vi "SPI Write Read N Frames.vi"(5 "CS Configuration":T1, 7 "SPI Channel (0)":u8, 8 "Error In":errorcluster, 9 "SPI Frame Size (0)":u8, 10 "Data":u8[](array[numeric]), 11 "LINX Resource":T3) -> (0 "Error Out":errorcluster, 1 "Read Data":u8[](array[numeric]), 3 "LINX Resource":T3)   [LabVIEW 2011, in "LVH-LINX.lvlib"]
doc: "Write/Read the specified SPI channel. SPI is full duplex, therefore the write and read operations take place simultaneously.\n\n<b>SPI Channel</b> specifies the device SPI channel to write/read to.\n\n<b>Data</b> is a U8 array of data bytes to shift out starting with Data[0] to Data[n-1].\n\n<b>SPI Frame Size</b> determinse the number of bytes shifted out between toggling CS.\n\n<b>CS Channel</b> is the Chip Select (DIO) channel to use during the SPI transaction.\n\n<b>CS Logic Level</b> specifies the logic level of the CS pin. Active low is most common and means that CS will idle high, then be driven low when a frame begins. The number of bytes specified in SPI Frame Size will be transfered, then CS will be driven high to end the frame. This process is repeated until all bytes in Data have been shifted out."
uses:
  LVH-LINX.lvlib
  Private/Type Defs/LINX Ref.ctl
  Private/Type Defs/Platform.ctl
  Private/Type Defs/Interface.ctl
  Private/Device/Type Defs/LINX Device Config.ctl
  Private/Device/Type Defs/TCP Config.ctl
  Private/Device/Type Defs/Channels.ctl
  SPI CS Config.ctl
  Private/Type Defs/Peripherals/SPI/SPI CS Logic Level.ctl
  Private/Type Defs/Peripheral.ctl
  Private/Type Defs/Channel FGV States.ctl
  Private/Device/Device.lvlib
  <vilib>/myRIO/Common/Instrument Driver Framework/myRIO v1.0/SPI/typedefs/SPI Frame Length.ctl
  <vilib>/myRIO/Common/Instrument Driver Framework/myRIO v1.0/SPI/typedefs/SPI Data Direction.ctl
  <vilib>/myRIO/Common/Instrument Driver Framework/myRIO v1.0/SPI/typedefs/SPI Clock Polarity.ctl
  <vilib>/LabVIEW Hacker/LINX/Private/Type Defs/Peripherals/SPI/SPI Clock Phase.ctl
  <vilib>/myRIO/Instrument Drivers/Onboard IO/SPI/typedefs/SPI Configuration.ctl
  <vilib>/myRIO/Common/Instrument Driver Framework/myRIO v1.0/SPI/typedefs/SPI Channels Enum.ctl
  <vilib>/myRIO/Common/Instrument Driver Framework/Utilities/typedefs/Generic FPGA Reference.ctl
  <vilib>/myRIO/Common/Instrument Driver Framework/Utilities/typedefs/myRIO v1.0 Reference.ctl
  <vilib>/myRIO/Common/Instrument Driver Framework/Utilities/typedefs/Hardware Version Enum.ctl
  <vilib>/myRIO/Common/Instrument Driver Framework/Utilities/typedefs/myRIO Generic Hardware Reference.ctl
  <vilib>/myRIO/Instrument Drivers/Onboard IO/SPI/typedefs/SPI Reference.ctl
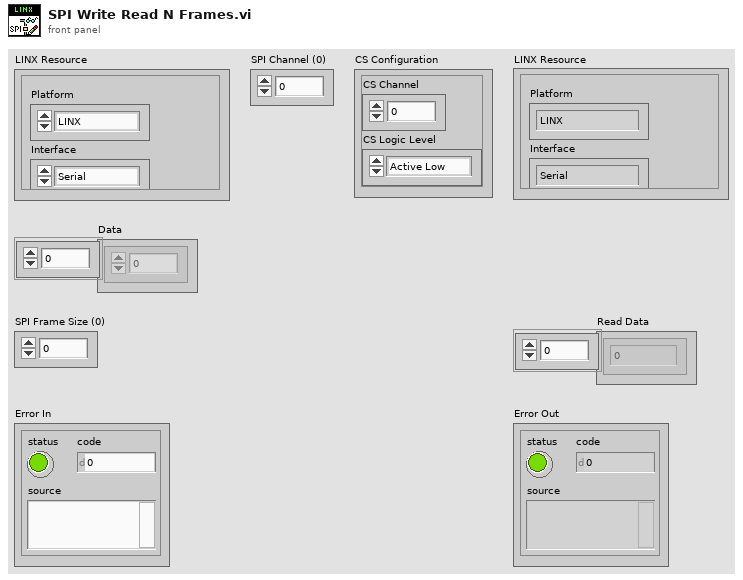
[diagram p1: front panel]
types:
  T1 = typedef "LVH-LINX.lvlib/SPI CS Config.ctl" = cluster{"CS Channel":u8, "CS Logic Level":T2}
  T2 = typedef "LVH-LINX.lvlib/SPI CS Logic Level.ctl" = enum8{"Active Low", "Active High"}
  T3 = typedef "LVH-LINX.lvlib/LINX Ref.ctl" = cluster{"Platform":T4, "Interface":T5, "LINX Device Config":T6}
  T4 = typedef "LVH-LINX.lvlib/Platform.ctl" = enum16{"LINX", "myRIO"}
  T5 = typedef "LVH-LINX.lvlib/Interface.ctl" = enum16{"Serial", "TCP"}
  T6 = typedef "LVH-LINX.lvlib/Device.lvlib/LINX Device Config.ctl" = cluster{"Interface":T5, "COM Port":refnum<visa-resource-name>, "TCP Configuration":T7, "Device Family":u8, "Device ID":u8, "Device Name":string, "TCP Ref":refnum<k5>, "Channels":T8}
  T7 = typedef "LVH-LINX.lvlib/Device.lvlib/TCP Config.ctl" = cluster{"IP Address":string, "Port":u16}
  T8 = typedef "LVH-LINX.lvlib/Channels.ctl" = cluster{"DI Channels":u8[], "DO Channels":u8[], "AI":u8[], "AO":u8[], "PWM":u8[], "QE":u8[], "UART":u8[], "I2C 2":u8[], "SPI":u8[], "CAN":u8[], "AI Ref (V)":dbl, "AO Resolution (Bits)":u8, "AO Ref (V)":dbl}
  T9 = typedef "LVH-LINX.lvlib/Peripheral.ctl" = enum8{"DI", "DO", "AI", "AO", "PWM", "QE", "UART", "I2C", "SPI", "CAN"}
  T10 = typedef "LVH-LINX.lvlib/Channel FGV States.ctl" = enum16{"Initialize", "Get", "Set"}
  T11 = typedef "SPI.lvlib/SPI Reference.ctl" = cluster{"myRIO Reference":T12, "SPI Channels Enum":T16, "SPI Configuration":T17}
  T12 = typedef "myRIO Generic Hardware Reference.ctl" = cluster{"myRIO Model":T13, "myRIO Hardware Reference":T14}
  T13 = typedef "Hardware Version Enum.ctl" = enum16{"Unknown", "myRIO-1900", "myRIO-1950"}
  T14 = typedef "myRIO v1.0 Reference.ctl" = cluster{"Generic FPGA Reference":T15, "Allow multiple opens":bool}
  T15 = typedef "Generic FPGA Reference.ctl" = refnum<k20>
  T16 = typedef "SPI Channels Enum.ctl" = enum16{"Not Connected", "A/SPI", "B/SPI"}
  T17 = typedef "SPI.lvlib/SPI Configuration.ctl" = cluster{"Frequency (Hz)":dbl, "Clock Phase":T18, "Clock Polarity":T19, "Data Direction":T20, "Frame Length":T21}
  T18 = typedef "LVH-LINX.lvlib/SPI Clock Phase.ctl" = enum8{"Leading", "Trailing"}
  T19 = typedef "SPI Clock Polarity.ctl" = enum8{"Low", "High"}
  T20 = typedef "SPI Data Direction.ctl" = enum8{"Most Significant Bit First", "Least Significant Bit First"}
  T21 = typedef "SPI Frame Length.ctl" = u8
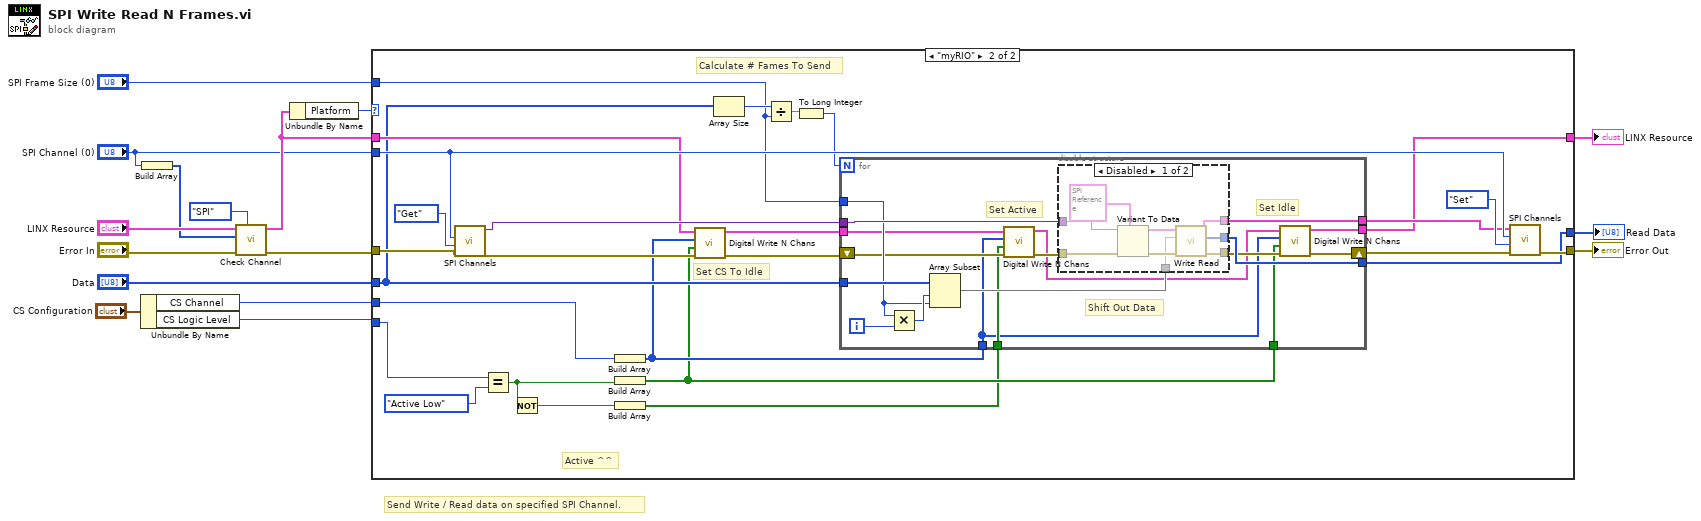
[diagram p0: block diagram]
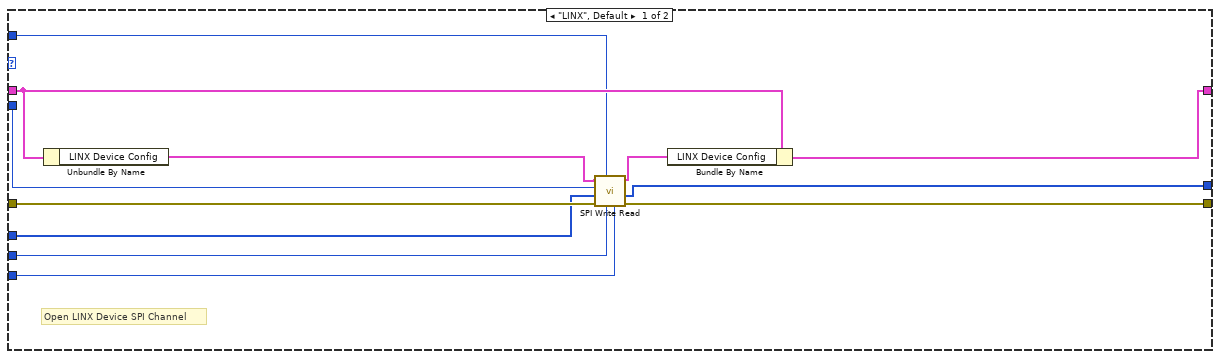
[diagram p2: hidden frame]
diagram:
  # "Send Write / Read data on specified SPI Channel."
  n1 = Unbundle By Name("CS Configuration") -> ("CS Channel"=w2:u8, "CS Logic Level"=w1:T2)
  n2 = Build Array("SPI Channel (0)") -> (w10:u8[])
  n3 = call "Check Channel.vi"("Peripheral"=Peripheral."SPI", "Error In"="Error In", "Channels"=w10, "LINX Resource"="LINX Resource") -> ("Error Out"=w11:errorcluster, "LINX Resource"=w12:T3)  [unwired: 5 in, 1 out]
  n4 = Unbundle By Name(w12) -> ("Platform"=w16:T4)
  n5 = case shown="\"myRIO\"" w16 {
    tunnel: w11 -> [w26 w53]
    tunnel: w12 -> [w28 w46]
    tunnel: [w27 w55] -> w15
    tunnel: [w17 w34] -> w4
    tunnel: "SPI Channel (0)" -> [w21 w52]
    tunnel: [w23 w47] -> w7
    tunnel: "Data" -> [w22 w41]
    tunnel: "SPI Frame Size (0)" -> [w20 w37]
    tunnel: w2 -> [w19 w33]
    tunnel: w1 -> [w18 w43]
    frame "LINX", Default {
      # "Open LINX Device SPI Channel"
      n6 = Unbundle By Name(w28) -> ("LINX Device Config"=w24:T6)
      n7 = call "SPI Write Read.vi"("CS Logic Level"=w18, "CS Pin (10)"=w19, "SPI Frame Size (1)"=w20, "Error In"=w26, "Data"=w22, "SPI Channel"=w21, "LINX Device Config"=w24) -> ("Error Out"=w27:errorcluster, "Read Data"=w23:u8[], "LINX Device Config"=w25:T6)  [unwired: 2 in]
      n8 = Bundle By Name(cluster=w28, "LINX Device Config"=w25) -> (w17:T3)
    }
    frame "myRIO" {
      # "Active ^^"
      # "Calculate # Fames To Send"
      # "Set CS To Idle"
      n9 = call "SPI Channels.vi"("Error In"=w53, "Channel State"=Channel_FGV_States."Get", "Channel Number"=w52) -> ("Error Out"=w45:errorcluster, "SPI Channel"=w48:variant)  [unwired: 7 in]
      n10 = Equal?(x=w43, y=SPI_CS_Logic_Level."Active Low") -> (x = y?=w32:bool)
      n11 = Not(x=w32) -> (.not. x?=w30:bool)
      n12 = Build Array(w33) -> (w35:u8[])
      n13 = Build Array(w32) -> (w31:bool[])
      n14 = Build Array(w30) -> (w29:bool[])
      n15 = call "Digital Write N Chans.vi"("Error In"=w45, "Values"=w31, "DO Channels"=w35, "LINX Resource"=w46) -> ("Error Out"=w44:errorcluster, "LINX Resource"=w36:T3)  [unwired: 6 in]
      n16 = Array Size(array=w41) -> (size(s)=w40:i32)
      n17 = Divide(x=w40, y=w37) -> (x/y=w39:dbl)
      n18 = To Long Integer(number=w39) -> (32bit integer=w38:i32)
      n19 = for {
        N: w38 -> [_]
        tunnel: [w73] -> w49
        tunnel: w48 -> [w72]
        tunnel: w41 -> [w70]
        tunnel: [w71] -> w47
        shift-right: [w62] -> w50
        shift-left: w44 -> [w65]
        tunnel: w37 -> [w66]
        tunnel: w36 -> [w63]
        tunnel: w35 -> [w56]
        tunnel: [w59] -> w34
        tunnel: w31 -> [w58]
        tunnel: w29 -> [w57]
        i -> [w68]
        # "Set Idle"
        # "Shift Out Data"
        # "Set Active"
        n20 = Multiply(x=w66, y=w68) -> (x*y=w67:i32)
        n21 = Array Subset(array=w70, index=w67, length=w66) -> (w69:u8[])
        n22 = call "Digital Write N Chans.vi"("Error In"=w65, "Values"=w57, "DO Channels"=w56, "LINX Resource"=w63) -> ("Error Out"=w64:errorcluster, "LINX Resource"=w60:T3)  [unwired: 6 in]
        n23 = disable-structure shown="Disabled" {
          disable-tunnel: [w80 _] -> w61
          disable-tunnel: w64 -> [w78 _]
          disable-tunnel: [w77 _] -> w73
          disable-tunnel: w72 -> [w76 _]
          disable-tunnel: w69 -> [w75 _]
          disable-tunnel: [w74 _] -> w71
          frame Disabled {
            n24 = Variant To Data(error in=w78, type=T11 {"myRIO Reference"={"myRIO Model"=enum."Unknown", "myRIO Hardware Reference"={"Generic FPGA Reference"=refnum, "Allow multiple opens"=FALSE}}, "SPI Channels Enum"=enum."Not Connected", "SPI Configuration"={"Frequency (Hz)"=0.0, "Clock Phase"=enum."Leading", "Clock Polarity"=enum."Low", "Data Direction"=enum."Most Significant Bit First", "Frame Length"=8}} ("SPI Ref In"), Variant=w76) -> (data=w81:T11, error out=w79:errorcluster)
            n25 = call <vilib>:"Write Read.vi"("error in (no error)"=w79, "Frames to Write"=w75, "SPI Ref In"=w81) -> ("error out"=w80:errorcluster, "Frames Read"=w74:u16[], "SPI Ref Out"=w77:T11)  [unwired: 6 in]
          }
          frame Enabled {
          }
        }
        n26 = call "Digital Write N Chans.vi"("Error In"=w61, "Values"=w58, "DO Channels"=w56, "LINX Resource"=w60) -> ("Error Out"=w62:errorcluster, "LINX Resource"=w59:T3)  [unwired: 6 in]
      }
      n27 = call "SPI Channels.vi"("Error In"=w50, "Channel State"=Channel_FGV_States."Set", "Channel Number"=w52, "SPI Channel"=w49) -> ("Error Out"=w55:errorcluster)  [unwired: 6 in, 1 out]
    }
  }
  "Error Out" <- w15
  "LINX Resource" <- w4
  "Read Data" <- w7
